vi "get_ini.vi"(4 "error out 3":errorcluster, 5 "Array":refnum<vi>[](array[refnum]), 6 "viName":string, 7 "Rgpn2._Application 2":refnum<k7>) -> (0 "error out":errorcluster, 2 "iniPath":path, 3 "Rgpn2._Application":refnum<k7>)   [LabVIEW 2010]
uses:
  <vilib>/Utility/config.llb/NI_LVConfig.lvlib
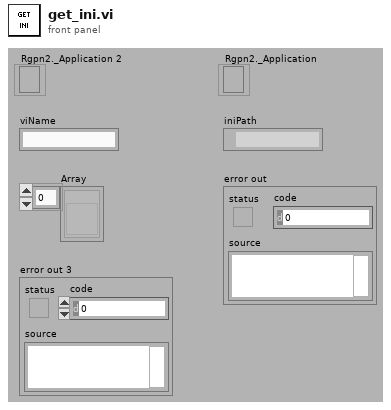
[diagram p1: front panel]
types:
  T1 = typedef "NI_LVConfig.lvlib/Config Data RefNum.ctl" = refnum<k1>
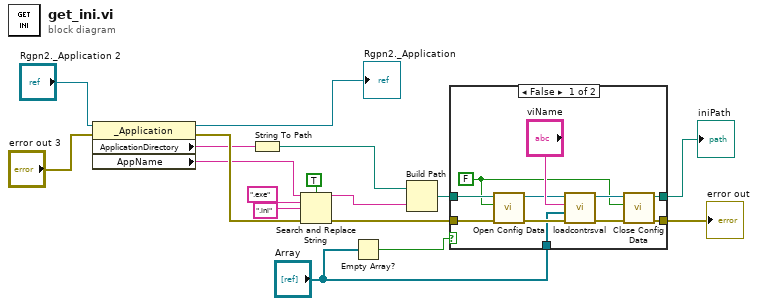
[diagram p0: block diagram]
diagram:
  n1 = property class="_Application"(reference="Rgpn2._Application 2", error in="error out 3") -> (reference out=→"Rgpn2._Application":refnum<k7>, error out=w15:errorcluster, "ApplicationDirectory"=w12:string, "AppName"=w13:string)
  n2 = String To Path(string=w12) -> (path=w4:path)
  n3 = Search and Replace String(case sensitive?=TRUE ("ignore case? (F)"), input string=w13, search string=".exe", replace string=".ini" ("replace string (\"\")"), error in=w15) -> (result string=w10:string, error out=w16:errorcluster)  [unwired: 3 in, 2 out]
  n4 = Empty Array?(array="Array") -> (empty?=w1:bool)
  n5 = Build Path(base path=w4, name or relative path=w10) -> (appended path=w11:path)
  n6 = case shown="False" w1 {
    tunnel: [w28 w29] -> w17
    tunnel: w16 -> [w27 w29]
    tunnel: w11 -> [w26 w30]
    tunnel: [w19 w30] -> w3
    tunnel: "Array" -> [w18 _]
    frame False {
      w20 = FALSE ("create file if necessary (T)")
      n7 = call <vilib>:"Open Config Data.vi"("error in (no error)"=w27, "create file if necessary (T)"=w20, "configuration file path"=w26) -> ("error out"=w22:errorcluster, "refnum"=w21:T1)  [unwired: 6 in, 1 out]
      n8 = call "loadcontrsval.vi"("error in"=w22, "Array"=w18, "Section"="viName", "refnum in"=w21) -> ("error out"=w24:errorcluster, "refnum out"=w23:T1)  [unwired: 1 in, 1 out]
      n9 = call <vilib>:"Close Config Data.vi"("error in (no error)"=w24, "write file if changed (T)"=w20, "refnum"=w23) -> ("error out"=w28:errorcluster, "file path"=w19:path)  [unwired: 7 in]
    }
    frame True {
    }
  }
  "error out" <- w17
  "iniPath" <- w3
